vi "Heat Exchangers.vi"(2 "Array In, M":dbl[](array[numeric]), 3 "input cluster, M":T1, 4 "input cluster, N":T1, 5 "Array In, N":dbl[](array[numeric])) -> (14 "MHX Heat Transfer (W)":dbl, 15 "NDHX Heating Transfer (W)":dbl, 16 "NDHX Tube Wall Temperature (K)":dbl, 17 "MHX Tube Wall Temperature (K)":dbl)   [LabVIEW 2019]
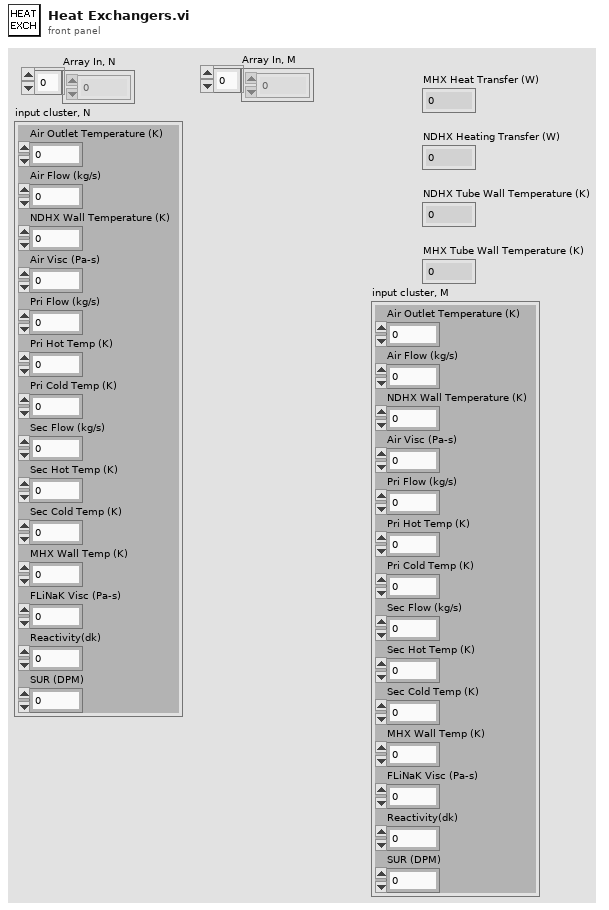
[diagram p1: front panel]
types:
  T1 = cluster{"Air Outlet Temperature (K)":dbl, "Air Flow (kg/s)":dbl, "NDHX Wall Temperature (K)":dbl, "Air Visc (Pa-s)":dbl, "Pri Flow (kg/s)":dbl, "Pri Hot Temp (K)":dbl, "Pri Cold Temp (K)":dbl, "Sec Flow (kg/s)":dbl, "Sec Hot Temp (K)":dbl, "Sec Cold Temp (K)":dbl, "MHX Wall Temp (K)":dbl, "FLiNaK Visc (Pa-s)":dbl, "Reactivity(dk)":dbl, "SUR (DPM)":dbl}
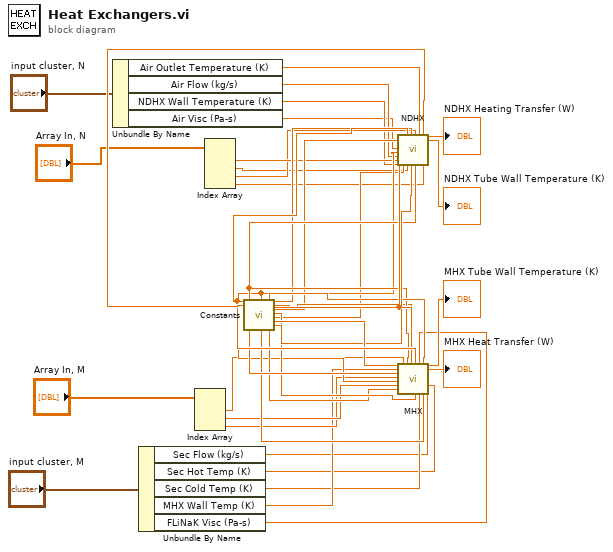
[diagram p0: block diagram]
diagram:
  n1 = Unbundle By Name("input cluster, N") -> ("Air Outlet Temperature (K)"=w5:dbl, "Air Flow (kg/s)"=w4:dbl, "NDHX Wall Temperature (K)"=w3:dbl, "Air Visc (Pa-s)"=w2:dbl)
  n2 = Unbundle By Name("input cluster, M") -> ("Sec Flow (kg/s)"=w7:dbl, "Sec Hot Temp (K)"=w8:dbl, "Sec Cold Temp (K)"=w9:dbl, "MHX Wall Temp (K)"=w10:dbl, "FLiNaK Visc (Pa-s)"=w11:dbl)
  n3 = Index Array(array="Array In, M") -> (element #1=w14:dbl, element #2=w13:dbl, element #3=w12:dbl)  [unwired: 3 in]
  n4 = Index Array(array="Array In, N") -> (element #1=w19:dbl, element #2=w17:dbl, element #3=w18:dbl, element #4=w16:dbl)  [unwired: 4 in]
  n5 = call "Constants.vi"() -> ("Cp of FLiNaK (J/kgK)"=w39:dbl, "Cp of Air (J/kgK)"=w40:dbl, "Thermal Conductivity of Hastealloy N (W/m-K)"=w28:dbl, "MHX Tube Diameter (m)"=w35:dbl, "Pipe Diameter (m)"=w33:dbl, "Thermal Conductivity of FLiNaK (W/m-K)"=w25:dbl, "MHX Length (m)"=w34:dbl, "Specific Heat Capacity of FLiBe (W/m-K)"=w30:dbl, "MHX Tube Wall Thickness (m)"=w27:dbl, "NDHX Tube Diameter (m)"=w24:dbl, "Thermal Conductivity of FLiBe (W/m-K)"=w26:dbl, "NDHX Tube Length (m)"=w23:dbl, "MHX Number of Tubes"=w31:dbl, "Stack Inner Diameter"=w21:dbl, "Pipe X-SectionArea (m^2)"=w36:dbl, "NDHX Number of Tubes"=w32:dbl)  [unwired: 5 in, 7 out]
  n6 = call "NDHX.vi"("NDHX Tube Length (m)"=w23, "Pipe Diameter (m)"=w33, "Air Average Viscosity (Pa-s)"=w2, "Thermal Conductivity of FLiNaK (W/m-K)"=w25, "Air Mass Flow (kg/s)"=w4, "Sec Hot Temp (K)"=w19, "NDHX Wall Temperature (K)"=w3, "Stack Inner Diameter (m)"=w21, "Cp of FLiNaK (J/kgK)"=w39, "Sec Cold Temp (K)"=w17, "NDHX Tube Diameter (m)"=w24, "NDHX Number of Tubes"=w32, "Air Cold Temperature (K)"=w18, "Thermal Conductivity of Hastealloy N (W/m-K)"=w28, "Air Hot Temperature (K)"=w5, "Cp of Air (J/kgK)"=w40, "Sec Mass Flow (kg/s)"=w16) -> ("NDHX Heating Transfer (W)"=→"NDHX Heating Transfer (W)":dbl, "Wall Temperature (K)"=→"NDHX Tube Wall Temperature (K)":dbl)  [unwired: 8 in, 1 out]
  n7 = call "MHX.vi"("Area"=w36, "MHX Tube Wall Temp"=w10, "MHX Tube Diameter"=w35, "Pri Cold Temp"=w12, "Thermal Conductivity of FLiNaK"=w25, "Pri Hot Temp"=w13, "MHX Tube Wall Thickness"=w27, "Pri Mass Flow"=w14, "Thermal Conductivity of Hastealloy N"=w28, "Thermal Conductivity of FLiBe"=w26, "Pipe Diameter"=w33, "Cp of FLiNaK"=w39, "MHX Number of Tubes"=w31, "FLiNaK Ave Viscosity"=w11, "Sec Cold Temp"=w9, "Specific Heat Capacity of FLiBe"=w30, "MHX Length"=w34, "Sec Hot Temp"=w8, "Sec Mass Flow"=w7) -> ("MHX Tube Wall Temperature (K)"=→"MHX Tube Wall Temperature (K)":dbl, "MHX Heat Transfer (W)"=→"MHX Heat Transfer (W)":dbl)  [unwired: 7 in]
